vi "GOOP_RenameClassControlLabel.vi"(7 "Label.Text":string, 8 "error in (no error)":errorcluster, 9 "Path":path, 10 "Typedef Path":path, 11 "GObject in":refnum<vi>) -> (0 "error out":errorcluster, 3 "Control out":refnum<vi>)   [LabVIEW 2020]
panel:
  out "NewLabelName":string
  out "name 2":string
  out "name":string
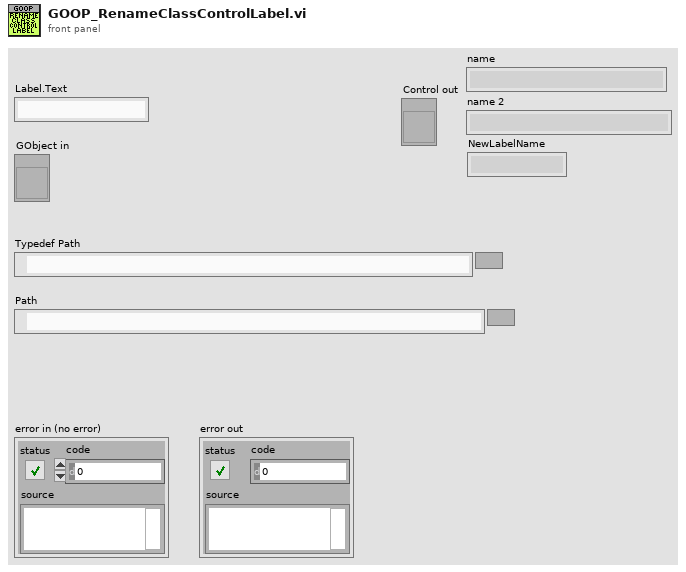
[diagram p1: front panel]
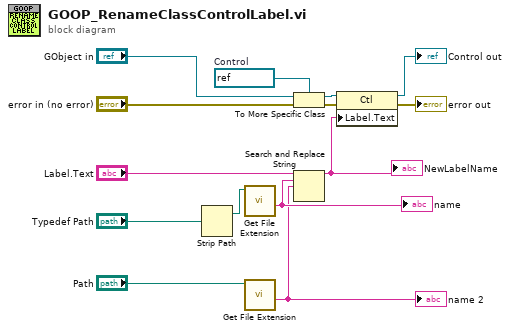
[diagram p0: block diagram]
diagram:
  w9 = refnum<vi> refnum  # Control
  n1 = Strip Path(path="Typedef Path") -> (stripped path=w5:path)  [unwired: 1 out]
  n2 = call <vilib>:"Get File Extension.vi"("file"=w5) -> ("filename without extension"=w3:string)  [unwired: 6 in, 4 out]
  "name" <- w3
  n3 = call <vilib>:"Get File Extension.vi"("file"="Path") -> ("filename without extension"=w2:string)  [unwired: 6 in, 4 out]
  "name 2" <- w2
  n4 = To More Specific Class(target class=w9, reference="GObject in", error in="error in (no error)") -> (specific class reference=w10:refnum<vi>, error out=w8:errorcluster)
  n5 = Search and Replace String(input string="Label.Text", search string=w3, replace string=w2) -> (result string=w1:string)  [unwired: 5 in, 3 out]
  "NewLabelName" <- w1
  n6 = property class="Ctl"(reference=w10, error in=w8, "Label.Text"=w1) -> (reference out=→"Control out":refnum<vi>, error out=→"error out":errorcluster)
